vi "No EOC Error.vi"(4 "error in (no error)":errorcluster) -> (1 "error out":errorcluster)   [LabVIEW 2015, in "NI_InternetTK_Common_VIs.lvlib"]
doc: "No EOC Error.vi checks to see if a connection closed error occurred and resets it to no error."
uses:
  NI_InternetTK_Common_VIs.lvlib
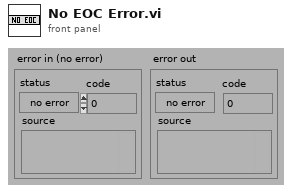
[diagram p1: front panel]
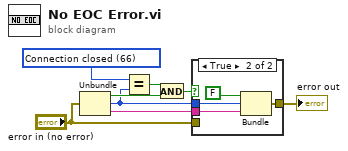
[diagram p0: block diagram]
diagram:
  w1 = u16 66 items=["No Error", "Argument Error", "Memory Full", "Out of Zone", "End of File", "File Already Open", "Generic File IO Error", "File Not Found", "File Permission Error", "Disk Full", "Duplicate Path", "Too Many Files Open", "Not Enabled", "Resource File Not Found", "Cannot Add Resource", "Resource Not Found", "Image Not Found", "Image Memory Error", "Pen Does Not Exist", "Config Bad Type", "Config Token Not Found", "Config Parse Error", "Config Memory Error", "Bad External Code Format", "Bad External Code Offset", "External Code Not Present", "Null Window", "Destroy Window Mixup", "Null Menu", "Print Aborted", "Bad Print Record", "Print Driver Error", "Windows Error During Print", "Memory Error During Print", "Print Dialog Error", "Generic Print Error", "Invalid Device Refnum", "Device Not Found", "Device Parameter Error", "Device Unit Error", "Can't Open Device", "Device Call Aborted", "Generic Error", "Cancelled By User", "Object ID Too Low", "Object ID Too High", "Object Not In Heap", "Unknown Heap", "Bad DefProc ID", "DefProc Not In Table", "Message Out Of Range", "Null Method", "Unknown Message", "Manager Call Not Supported", "Bad address", "Connection In progress", "Connection timed out", "Connection is already in progress", "Network attribute not supported", "Network error", "Address in use", "System out of memory", "Connection aborted", "Connection refused", "Connection is not connected", "Connection is already connected", "Connection closed", "Initialize error (interapplication manager)", "Bad occurrence", "Wait on unbound occurrence handler", "Occurrence queue overflow", "Bad path", "Semaphore not signaled", "Unrecognized type (interapplication manager)"]
  n1 = Unbundle("error in (no error)") -> ("status"=w7:bool, "code"=w3:i32, "source"=w4:string)
  n2 = Equal?(x=w1, y=w3) -> (x = y?=w6:bool)
  n3 = And(x=w6, y=w7) -> (x .and. y?=w5:bool)
  n4 = case shown="True" w5 {
    tunnel: "error in (no error)" -> [w9 _]
    tunnel: [w9 w13] -> w2
    tunnel: w4 -> [_ w12]
    tunnel: w3 -> [_ w11]
    frame False {
    }
    frame True {
      n5 = Bundle(FALSE, "code"=w11, "source"=w12) -> (w13:cluster{bool, "code":i32, "source":string})  [unwired: 1 out]
    }
  }
  "error out" <- w2
